vi "18_TCP_READ_write_OLD.vi"() -> ()   [LabVIEW 2019]
panel:
  out "concatenated string":string
  out "decimal integer string 3":string
  out "number 4":u32
  out "substring 3":string
  out "decimal integer string 4":string
  out "number 5":u32
  out "substring 4":string
  out "decimal integer string 2":string
  out "number 3":u32
  out "substring 2":string
  out "decimal integer string":string
  out "number 2":u32
  out "substring":string
  out "hex integer string":string
  out "net address":u32
  out "data out":string
  out "remote address":string
  out "remote port":u16
  in  "bytes to read":i32
  out "listener ID":refnum<k5>
  out "message":string=" INSTRUCTIONS:\r\rNormal Use:  When using subVIs that incorporate the error in/error out (or error I/O) structure, place this handler where you want to inform the user of an error, typically at the end of the I/O data path, as the last action of the program.  If the error in error? is ERROR, the handler creates a message describing the error and its source.  If the type of dialog = 1 (default), the message is displayed to the user, who can only acknowedge it.  If the type = 2, the user can acknowledge the message or abort execution; aborting a program with active I/O is not recommended.  If the type = 0, no message is displayed; this is used to process the error programmatically, and the error out cluster elements are wired to individual terminals for that reason.  \r\rOther Use:\n\r\nlocal testing.  To test the error code of a subVI or function that does not have the error I/O structure, you can wire its error code and a source string to the local error code and error source inputs.  If error in error? indicates no error and error code is not equal to 0, the local code and source are substituted for the error in values, and error? is set TRUE (ERROR)."
  out "data out 2":string
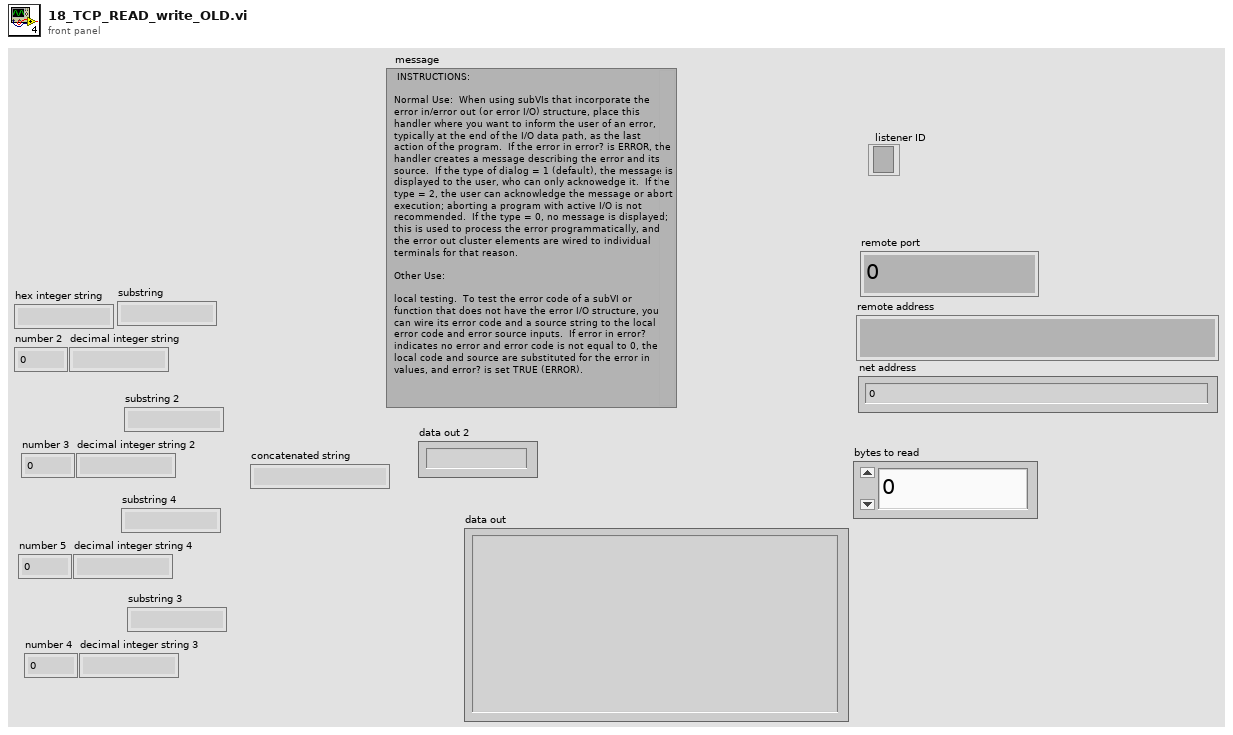
[diagram p1: front panel]
types:
  T1 = enum16{"Standard", "Buffered", "CRLF", "Immediate"}
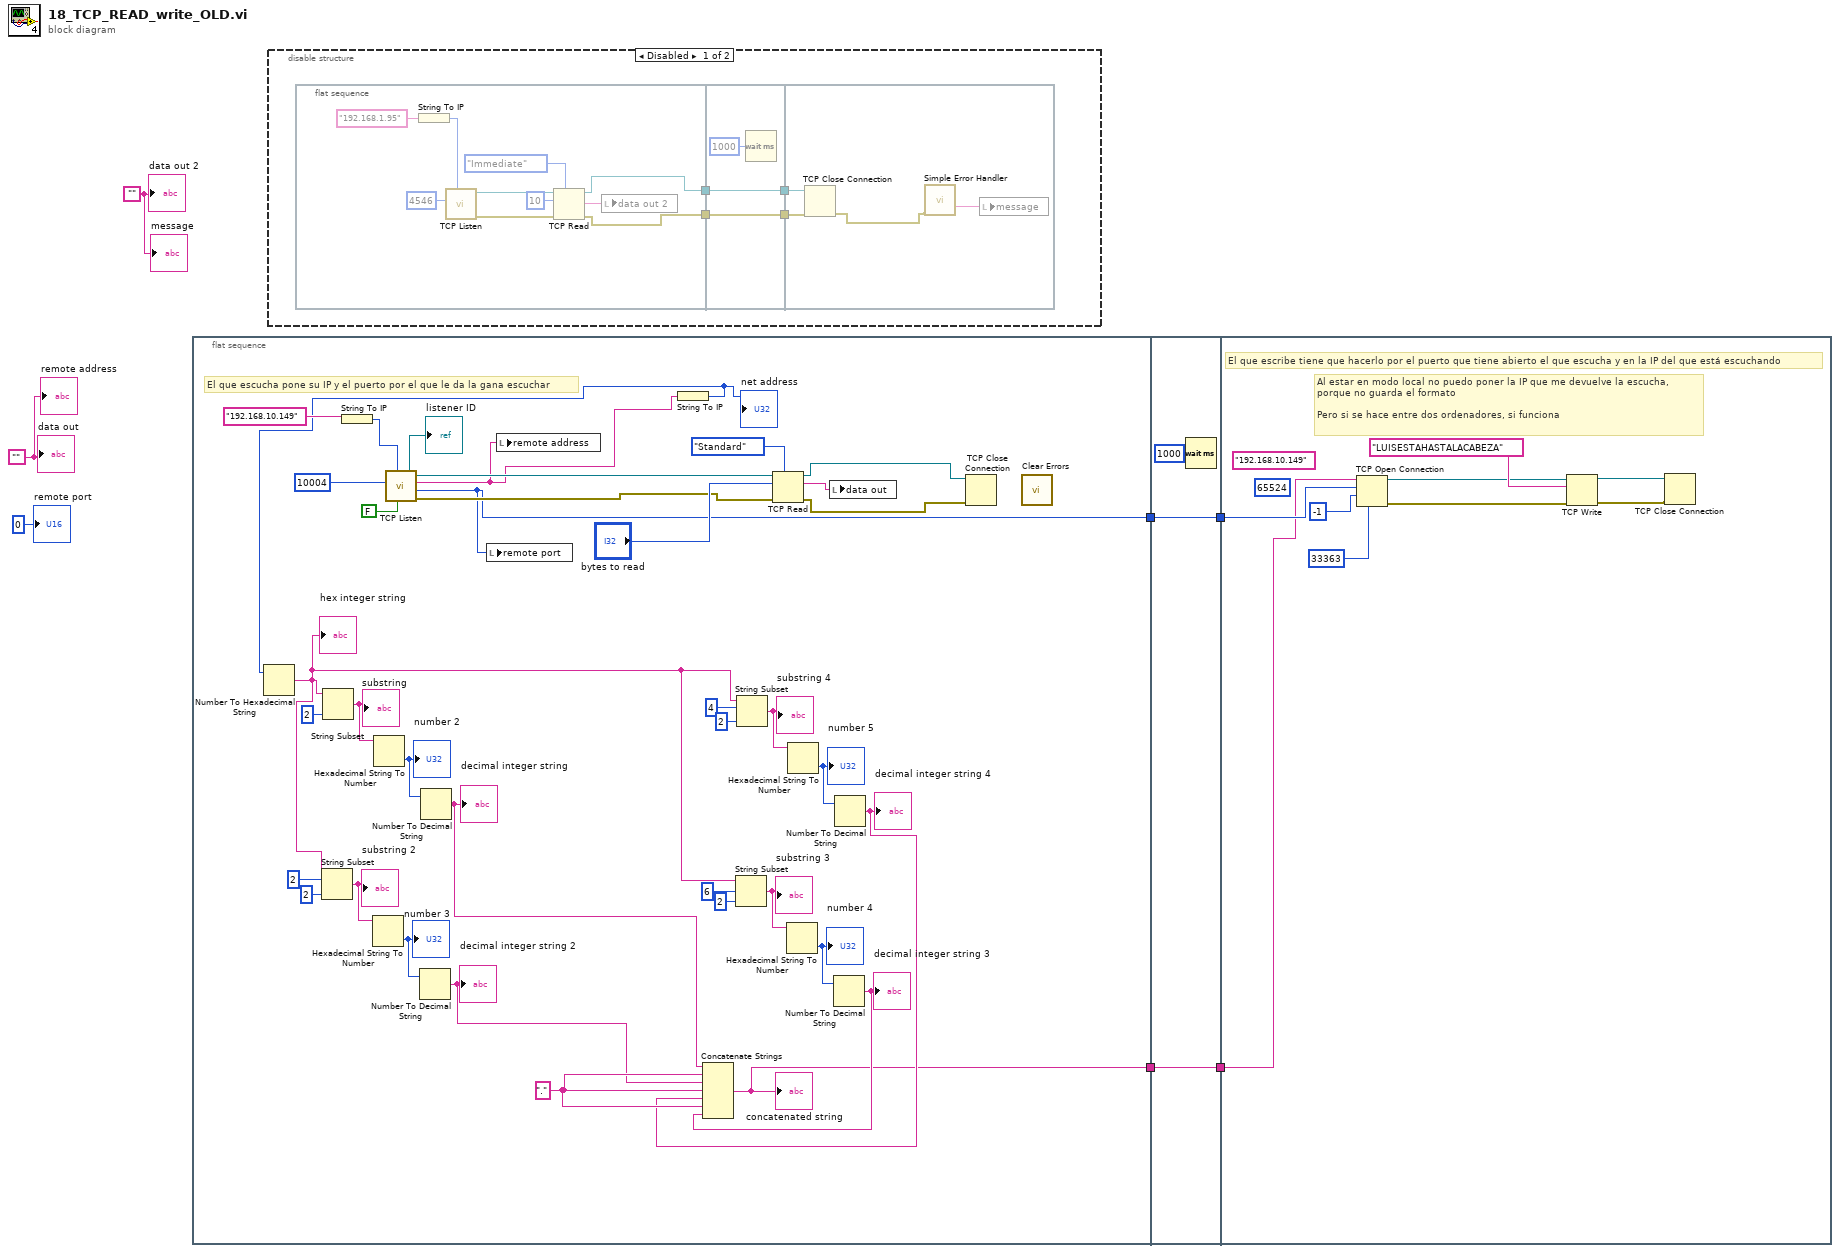
[diagram p0: block diagram]
diagram:
  w4 = ""
  w7 = ""
  n1 = flat-sequence {
    tunnel: [w31] -> w5
    tunnel: [w8] -> w1
    tunnel: [w46] -> w6
    tunnel: w5 -> [w46]
    tunnel: [w45] -> w2
    tunnel: w1 -> [w45]
    tunnel: w6 -> [w49]
    tunnel: w2 -> [w48]
    frame #0 {
      w14 = "."
      # "El que escucha pone su IP y el puerto por el que le da la gana escuchar"
      n2 = String To IP(1:"192.168.10.149") -> (0:w42:u32)
      n3 = call <vilib>:"TCP Listen.vi"("resolve remote address (T)"=FALSE, "net address"=w42, "port"=u16 10004) -> ("error out"=w38:errorcluster, "remote port"=w31:u16, "remote address"=w32:string, "connection ID"=w40:refnum<k5>, "listener ID"=→"listener ID":refnum<k5>)  [unwired: 4 in]
      n4 = local write "remote port"(w31) -> ()
      n5 = local write "remote address"(w32) -> ()
      n6 = String To IP(1:w32) -> (0:w9:u32)
      "net address" <- w9
      n7 = Number To Hexadecimal String(2:w9) -> (0:w18:string)  [unwired: 1 in]
      "hex integer string" <- w18
      n8 = String Subset(string=w18, offset (0)=2, length (rest)=2 ("length (rest)")) -> (substring=w26:string)
      "substring 2" <- w26
      n9 = String Subset(string=w18, length (rest)=2 ("length (rest)")) -> (substring=w29:string)  [unwired: 1 in]
      "substring" <- w29
      n10 = Hexadecimal String To Number(string=w26) -> (number=w27:u32)  [unwired: 2 in, 1 out]
      "number 3" <- w27
      n11 = Hexadecimal String To Number(string=w29) -> (number=w28:u32)  [unwired: 2 in, 1 out]
      "number 2" <- w28
      n12 = Number To Decimal String(number=w27) -> (decimal integer string=w12:string)  [unwired: 1 in]
      "decimal integer string 2" <- w12
      n13 = Number To Decimal String(number=w28) -> (decimal integer string=w13:string)  [unwired: 1 in]
      "decimal integer string" <- w13
      n14 = String Subset(string=w18, offset (0)=6, length (rest)=2 ("length (rest)")) -> (substring=w23:string)
      "substring 3" <- w23
      n15 = String Subset(string=w18, offset (0)=4, length (rest)=2 ("length (rest)")) -> (substring=w20:string)
      "substring 4" <- w20
      n16 = TCP Read(connection ID=w40, bytes to read="bytes to read", error in (no error)=w38, 7:T1."Standard" ("mode (standard)")) -> (connection ID out=w35:refnum<k5>, data out=w36:string, error out=w34:errorcluster)  [unwired: 1 in]
      n17 = Hexadecimal String To Number(string=w23) -> (number=w22:u32)  [unwired: 2 in, 1 out]
      "number 4" <- w22
      n18 = Hexadecimal String To Number(string=w20) -> (number=w21:u32)  [unwired: 2 in, 1 out]
      "number 5" <- w21
      n19 = local write "data out"(w36) -> ()
      n20 = Number To Decimal String(number=w22) -> (decimal integer string=w10:string)  [unwired: 1 in]
      "decimal integer string 3" <- w10
      n21 = Number To Decimal String(number=w21) -> (decimal integer string=w11:string)  [unwired: 1 in]
      "decimal integer string 4" <- w11
      n22 = Concatenate Strings(w13, w14, w12, w14, w11, w14, w10) -> (w8:string)
      "concatenated string" <- w8
      n23 = TCP Close Connection(connection ID=w35, error in (no error)=w34) -> ()  [unwired: 1 in, 2 out]
      n24 = call <vilib>:"Clear Errors.vi"() -> ()  [unwired: 6 in, 2 out]
    }
    frame #1 {
      n25 = Wait (ms)(milliseconds to wait=u32 1000) -> ()  [unwired: 1 out]
    }
    frame #2 {
      (unwired) u16 65524 ("remote port or service name")
      (unwired) "192.168.10.149" ("address")
      # "El que escribe tiene que hacerlo por el puerto que tiene abierto el que escucha y en la IP del que está escuchando"
      # "Al estar en modo local no puedo poner la IP que me devuelve la escucha,\nporque no guarda el formato \n\nPero si se hace entre dos ordenadores, si funciona"
      n26 = TCP Open Connection(address=w48, remote port or service name=w49, timeout ms (60000)=-1, local port=u16 33363 ("local port (0)")) -> (connection ID=w52:refnum<k5>, error out=w54:errorcluster)  [unwired: 1 in]
      n27 = TCP Write(connection ID=w52, data in="LUISESTAHASTALACABEZA", error in (no error)=w54) -> (connection ID out=w50:refnum<k5>, error out=w51:errorcluster)  [unwired: 1 in, 1 out]
      n28 = TCP Close Connection(connection ID=w50, error in (no error)=w51) -> ()  [unwired: 1 in, 2 out]
    }
  }
  n29 = disable-structure shown="Disabled" {
    frame Disabled {
      n30 = flat-sequence {
        tunnel: [w69] -> w60
        tunnel: [w67] -> w59
        tunnel: w60 -> [w73]
        tunnel: w59 -> [w72]
        tunnel: [w73] -> w58
        tunnel: [w72] -> w57
        tunnel: w58 -> [w75]
        tunnel: w57 -> [w74]
        frame #0 {
          n31 = String To IP(1:"192.168.1.95" ("name")) -> (0:w63:u32)
          n32 = call <vilib>:"TCP Listen.vi"("net address"=w63, "port"=u16 4546) -> ("error out"=w68:errorcluster, "connection ID"=w64:refnum<k5>)  [unwired: 5 in, 3 out]
          n33 = TCP Read(connection ID=w64, bytes to read=10, error in (no error)=w68, 7:T1."Immediate" ("mode (standard)")) -> (connection ID out=w69:refnum<k5>, data out=w61:string, error out=w67:errorcluster)  [unwired: 1 in]
          n34 = local write "data out 2"(w61) -> ()
        }
        frame #1 {
          n35 = Wait (ms)(milliseconds to wait=u32 1000) -> ()  [unwired: 1 out]
        }
        frame #2 {
          n36 = TCP Close Connection(connection ID=w75, error in (no error)=w74) -> (error out=w77:errorcluster)  [unwired: 1 in, 1 out]
          n37 = call <vilib>:"Simple Error Handler.vi"("error in (no error)"=w77) -> ("source out"=w76:string)  [unwired: 4 in, 4 out]
          n38 = local write "message"(w76) -> ()
        }
      }
    }
    frame Enabled {
    }
  }
  "data out 2" <- w7
  "message" <- w7
  "data out" <- w4
  "remote address" <- w4
  "remote port" <- u16 0 ("remote port")
